vi "SoundAcqGen.vi"() -> ()   [LabVIEW 2017]
uses:
  <vilib>/Analysis/4window.llb/windowTd.ctl
  <vilib>/sound2/lvsound2.llb/Sampling Mode.ctl
  <vilib>/sound2/lvsound2.llb/Sound Data Format.ctl
  <extravilib>/ChannelInstances/Stream-a[.](wfm(dbl))/Read With Abort.vi
  <extravilib>/ChannelInstances/Stream-a[.](wfm(dbl))/Write With Abort.vi
  <extravilib>/ChannelInstances/Stream-a[.](wfm(dbl))/EndpointRead.vi
  <extravilib>/ChannelInstances/Stream-a[.](wfm(dbl))/Endpoint.vi
  <extravilib>/ChannelInstances/Stream-a[.](wfm(dbl))/Instantiate.vi
  <extravilib>/ChannelInstances/Stream-a[.](wfm(dbl))/)Channel.vi
  <resource>/ChannelSupport/_ChannelSupport/WaitIfNeeded.vi
  <vilib>/measure/maspectr.llb/FFT Power Spectrum and PSD for N Chan.vi
  <vilib>/sound2/lvsound2.llb/Sound Input Read (DBL).vi
  <vilib>/measure/NI_MAPro.lvlib
  <extravilib>/ChannelInstances/Stream-a[.](wfm(dbl)).lvlib
  <vilib>/Analysis/NI_AALPro.lvlib
panel:
  in  "window":T1=1 items=["Rectangle"=0, "Hanning"=1, "Hamming"=2, "Blackman-Harris"=3, "Exact Blackman"=4, "Blackman"=5, "Flat Top"=6, "4 Term B-Harris "=7, "7 Term B-Harris"=8, "Low Sidelobe"=9, "Blackman Nuttall"=11, "Triangle"=30, "Bartlett-Hanning"=31, "Bohman"=32, "Parzen"=33, "Welch"=34, "Kaiser"=60, "Dolph-Chebyshev"=61, "Gaussian"=62]
  in  "dB On (F)":bool
  out "Spectrum":cluster{"f0":dbl, "df":dbl, "magnitude":dbl[]}[](graph)
  in  "number of samples/ch":i32=10000
  in  "stop":bool
  out "Waveform Graph":waveform(dbl)[](graph)
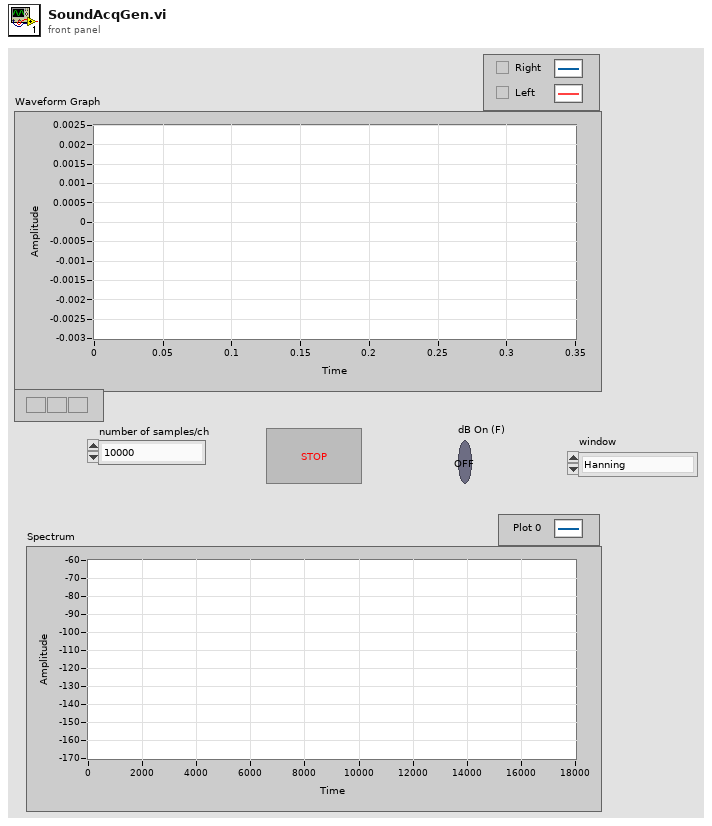
[diagram p1: front panel]
types:
  T1 = typedef "NI_AALPro.lvlib/windowTd.ctl" = u32
  T2 = typedef "Sound Data Format.ctl" = cluster{"sample rate (S/s)":dbl, "number of channels":i32, "bits per sample":i32}
  T3 = typedef "Sampling Mode.ctl" = i32
  T4 = typedef "Sound Input Task ID.ctl" = u32
  T5 = typedef "Stream-a[.](wfm(dbl)).lvlib/)Channel.ctl" = refnum<queue>
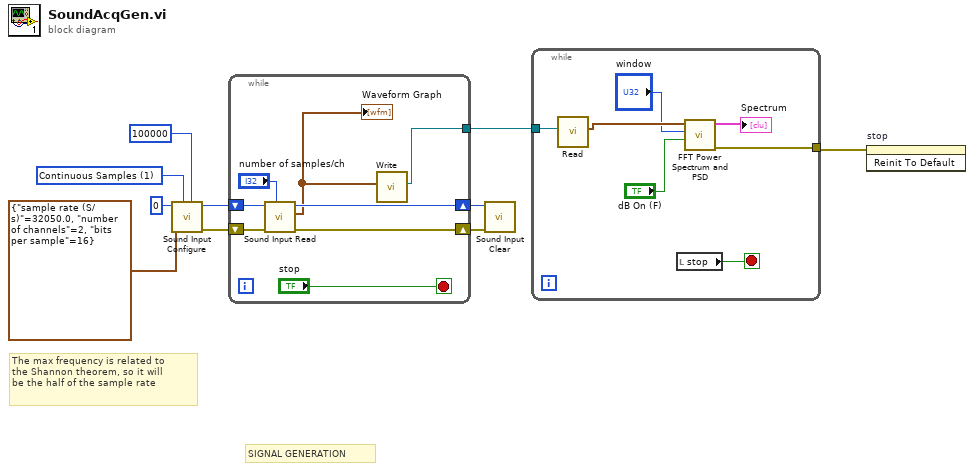
[diagram p0: block diagram]
diagram:
  w9 = T3 1 items=["Finite Samples", "Continuous Samples"] ("sample mode")
  # "SIGNAL GENERATION"
  # "The max frequency is related to\nthe Shannon theorem, so it will\nbe the half of the sample rate"
  n1 = call <vilib>:"Sound Input Configure.vi"("number of samples/ch"=100000, "sample mode"=w9, "sound format"=T2 {"sample rate (S/s)"=32050.0, "number of channels"=2, "bits per sample"=16}, "device ID"=u32 0) -> ("error out"=w6:errorcluster, "task ID"=w5:T4)  [unwired: 6 in]
  n2 = while {
    shift-right: [w16] -> w4
    shift-left: w6 -> [w18]
    shift-right: [w15] -> w3
    shift-left: w5 -> [w17]
    tunnel: [w11] -> w1
    stop <- "stop" stop-if-true
    n3 = call-poly <vilib>:"Sound Input Read.vi"("number of samples/ch"="number of samples/ch", "error in (no error)"=w18, "task ID"=w17) -> ("error out"=w16:errorcluster, "data"=w12:waveform(dbl)[], "task ID out"=w15:T4)  [unwired: 6 in]
    "Waveform Graph" <- w12
    n4 = call <extravilib>:"Write.vi"("element"=w12) -> ("channel"=w11:T5)  [unwired: 8 in, 2 out]
  }
  n5 = call <vilib>:"Sound Input Clear.vi"("error in (no error)"=w4, "task ID"=w3) -> ()  [unwired: 9 in, 1 out]
  n6 = while {
    tunnel: [w23] -> w2
    tunnel: w1 -> [w22]
    stop <- w25 stop-if-true
    n7 = call <extravilib>:"Read.vi"("channel"=w22) -> ("element"=w21:waveform(dbl)[])  [unwired: 6 in, 4 out]
    n8 = local read "stop"() -> (w25:bool)
    n9 = call-poly <vilib>:"FFT Power Spectrum and PSD.vi"("dB On (F)"="dB On (F)", "window"="window", "time signals"=w21) -> ("error out"=w23:errorcluster, "Power Spectrum / PSD"=→"Spectrum":cluster{"f0":dbl, "df":dbl, "magnitude":dbl[]}[])  [unwired: 5 in, 2 out]
  }
  n10 = invoke on="stop" class="Bool (strict)" method="Reinit To Default"(error in=w2) -> ()  [unwired: 2 in, 3 out]
